vi "Init IO.vi"   [LabVIEW 2019, in "HD44780.lvlib"]
uses:
  HD44780.lvlib
  <vilib>/rvi/eio/common/nirviEmuTemplateMethod_errors.vi
  <vilib>/eio/EIOMethodNode/EIOMethodNode.xnode
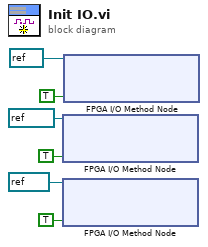
[diagram p0: block diagram]
diagram:
  n1 = xnode "FPGA I/O Method Node"("FPGA I/O In"=refnum<k21> "RW", "Enable"=TRUE) -> ()  [unwired: 1 out]
  n2 = xnode "FPGA I/O Method Node"("FPGA I/O In"=refnum<k21> "RS", "Enable"=TRUE) -> ()  [unwired: 1 out]
  n3 = xnode "FPGA I/O Method Node"("FPGA I/O In"=refnum<k21> "E", "Enable"=TRUE) -> ()  [unwired: 1 out]
